vi "Variant_FormatToString.vi"(7 "Formatter":refnum<class "StringFormatter.lvclass">, 10 "Variant":variant) -> (2 "Value":string)   [LabVIEW 2013, in "OpenVariant.lvlib"]
uses:
  OpenVariant.lvlib
  StringFormatter/StringFormatter.lvclass
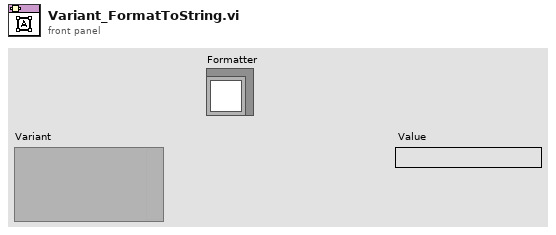
[diagram p1: front panel]
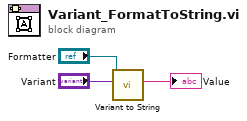
[diagram p0: block diagram]
diagram:
  n1 = call "Variant to String.vi"("Variant"="Variant", "StringFormatter in"="Formatter") -> ("Value"=→"Value":string)  [unwired: 7 in, 2 out]
